vi "read field.vi"(8 "error in":errorcluster, 11 "Varian Magnet.lvclass":refnum<class "Varian Magnet.lvclass">) -> (0 "error out":errorcluster, 2 "Current field (T)":dbl[unit], 3 "Varian Magnet.lvclass 2":refnum<class "Varian Magnet.lvclass">)   [LabVIEW 2009, in "Varian Magnet.lvclass"]
uses:
  Varian Magnet.lvclass
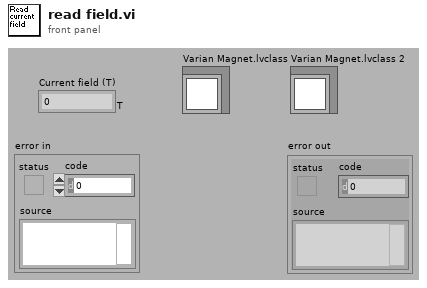
[diagram p1: front panel]
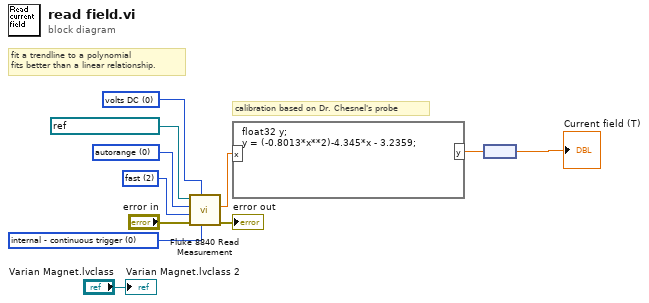
[diagram p0: block diagram]
diagram:
  w5 = u16 0 items=["volts DC", "volts AC", "2-wire k.ohms", "4-wire k.ohms", "mA DC", "mA AC"] ("function (0:volts DC)")
  w11 = u16 0 items=["internal - continuous trigger", "external - rear panel trigger with delay", "external - bus trigger with delay", "external - rear panel trigger", "external - bus trigger"] ("trigger mode (0:internal)")
  w10 = u16 2 items=["slow", "medium", "fast"] ("rate (0:slow)")
  w9 = u16 0 items=["autorange", "200mV, 200 ohms", "2V, 2 kohms", "20V, 20 kohms", "200V, 200 kohms", "1000Vdc, 700 Vac, 2 Mohms", "20 Mohms"] ("range (0:auto)")
  # "calibration based on Dr. Chesnel's probe"
  # "fit a trendline to a polynomial\nfits better than a linear relationship."
  n1 = call "Fluke 8840 Read Measurement.vi"("trigger mode (0:internal)"=w11, "function (0:volts DC)"=w5, "error in (no error)"="error in", "rate (0:slow)"=w10, "range (0:auto)"=w9, "VISA resource name"=refnum<visa-resource-name> "GPIB0::2::INSTR") -> ("error out"=→"error out":errorcluster, "measurement"=w2:dbl)  [unwired: 4 out]
  n2 = formula code="float32 y;\ny = (-0.8013*x**2)-4.345*x - 3.2359;"("x"=w2) -> ("y"=w1:sgl)
  n3 = node(w1) -> (→"Current field (T)":sgl[unit])
  "Varian Magnet.lvclass 2" <- "Varian Magnet.lvclass"
